vi "test Encode Parameters into Words for Labels in a Channel.vi"(8 "error in":errorcluster, 11 "TestCase in":refnum<class "Engine.lvclass">) -> (0 "error out":errorcluster, 3 "TestCase out":refnum<class "Engine.lvclass">)   [LabVIEW 2020, in "Engine.lvclass"]
uses:
  Engine.lvclass
  Shared/RT Label Settings.ctl
  Shared/Label.ctl
  Shared/RT Parameters.ctl
  Shared/Parameter Definition.ctl
  <vilib>/NI/NI VeriStand Encoding and Decoding/Encoding.ctl
  <vilib>/NI VeriStand/Custom Device API/Custom Device Item Ref.ctl
  Shared/Transfer Type.ctl
  <vilib>/NI VeriStand/Custom Device API/Data Reference.ctl
  <vilib>/addons/_JKI Toolkits/VI Tester/TestCase.llb/TestCase.lvclass
  <vilib>/NI VeriStand/Custom Device API/Custom Device API.lvlib
  <vilib>/NI/NI VeriStand Encoding and Decoding/Encoding and Decoding.lvlib
  Engine/Implementation/Tx Scheduled Labels Execution Unit/Tx Scheduled Labels Execution Unit.lvclass
  C:/Program Files (x86)/National Instruments/LabVIEW 2020/vi.lib/addons/_JKI Toolkits/VI Tester/TestCase.llb/TestCase.lvclass
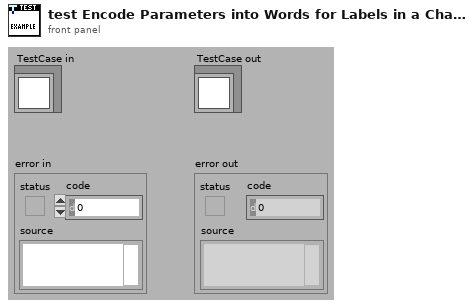
[diagram p1: front panel]
types:
  T1 = typedef "RT Label Settings.ctl" = cluster{"Name":string, "xmlName":string, "label":T2, "transfer period":u32, "SDI_Enabled":bool, "SDI":u8, "parameter driver data":T3, "transfer type":T7, "has timestamp?":bool, "Label Disable/Trigger Channel Reference":T6, "Message Handle":u64, "Initialized?":bool, "Word Initial Raw Value":u32, "Label Timestamp Channel Data Reference":T8, "disabled":bool}
  T2 = typedef "Label.ctl" = u8
  T3 = typedef "RT Parameters.ctl" = cluster{"parameter definitions":T4[], "Tx parameter refs":T6[]}
  T4 = typedef "Parameter Definition.ctl" = cluster{"start index":i32, "size":i32, "encoding":T5, "signed":bool, "scale multiplier":dbl, "scale offset":dbl, "default value":dbl}
  T5 = typedef "Encoding and Decoding.lvlib/Encoding.ctl" = enum16{"BNR", "BCD", "Discrete"}
  T6 = typedef "Custom Device API.lvlib/Custom Device Item Ref.ctl" = u64
  T7 = typedef "Transfer Type.ctl" = enum16{"Scheduled", "Acyclic", "Block", "Strobe"}
  T8 = typedef "Custom Device API.lvlib/Data Reference.ctl" = i32
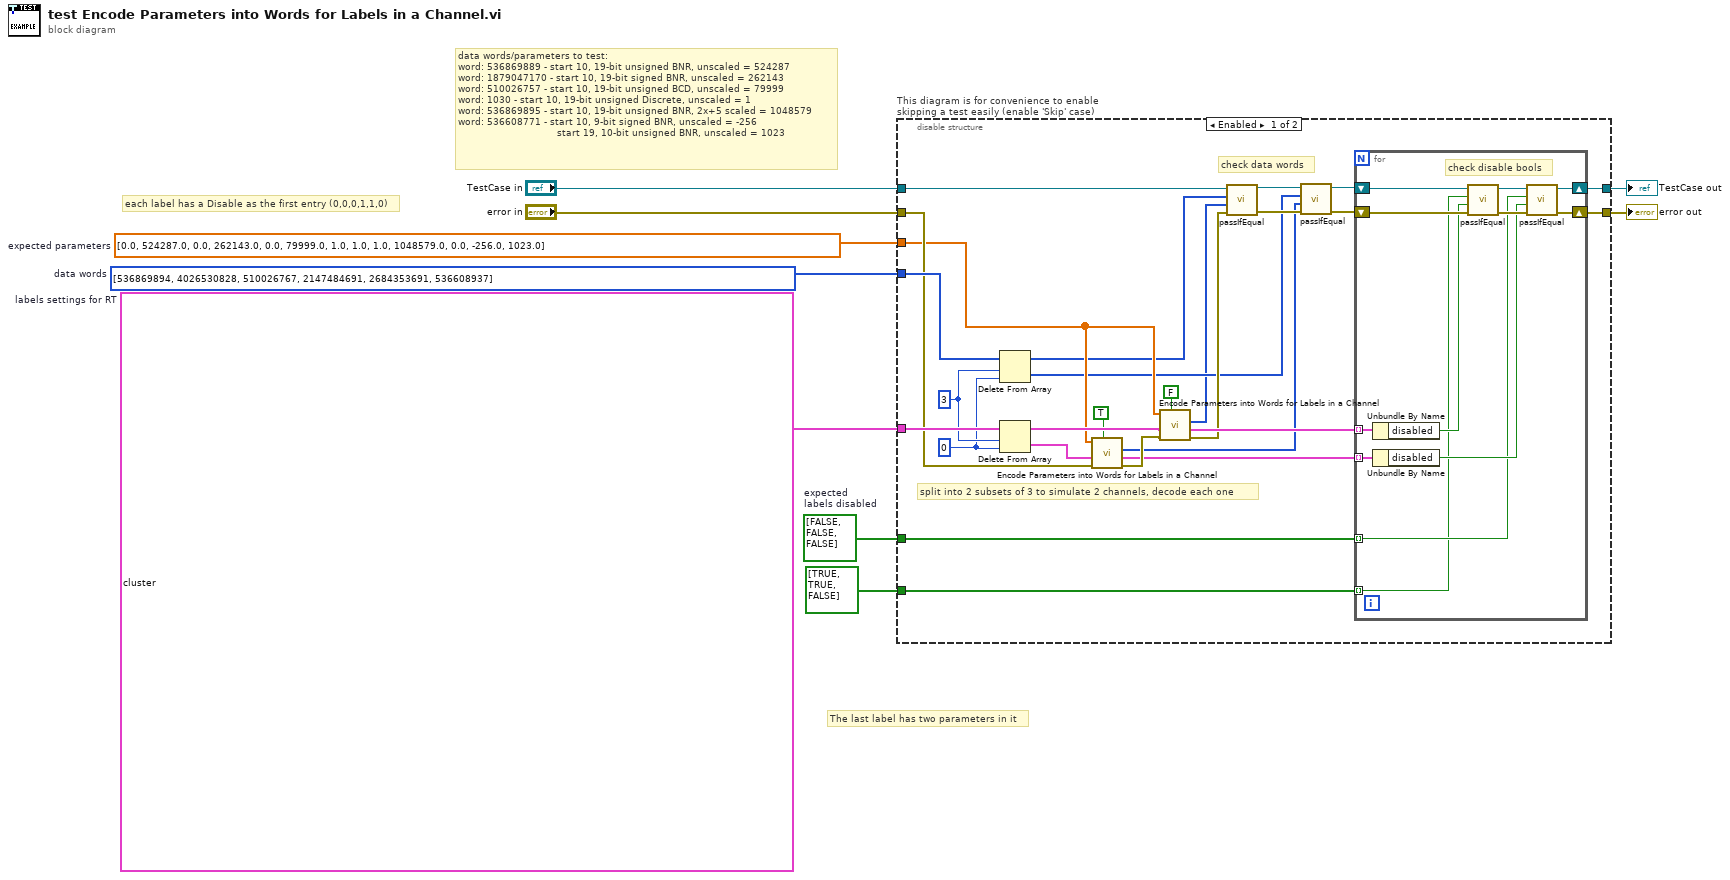
[diagram p0: block diagram]
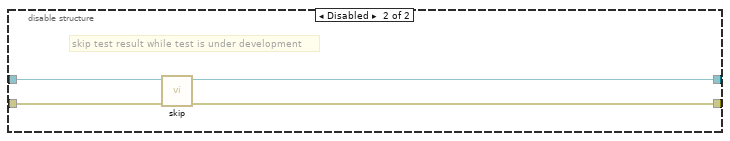
[diagram p2: hidden frame]
diagram:
  w2 = bool[] [FALSE, FALSE, FALSE]  # expected labels disabled
  w4 = dbl[] [0.0, 524287.0, 0.0, 262143.0, 0.0, 79999.0, 1.0, 1.0, 1.0, 1048579.0, 0.0, -256.0, 1023.0]  # expected parameters
  w5 = T1[] [{"Name"="", "xmlName"="", "label"=6, "transfer period"=10, "SDI_Enabled"=FALSE, "SDI"=0, "parameter driver data"={"parameter definitions"=[{"start index"=10, "size"=19, "encoding"=enum."BNR", "signed"=FALSE, "scale multiplier"=1.0, "scale offset"=0.0, "default value"=0.0}], "Tx parameter refs"=[]}, "transfer type"=enum."Scheduled", "has timestamp?"=FALSE, "Label Disable/Trigger Channel Reference"=0, "Message Handle"=0, "Initialized?"=FALSE, "Word Initial Raw Value"=0, "Label Timestamp Channel Data Reference"=0, "disabled"=FALSE}, {"Name"="", "xmlName"="", "label"=12, "transfer period"=10, "SDI_Enabled"=FALSE, "SDI"=0, "parameter driver data"={"parameter definitions"=[{"start index"=10, "size"=19, "encoding"=enum."BNR", "signed"=TRUE, "scale multiplier"=1.0, "scale offset"=0.0, "default value"=0.0}], "Tx parameter refs"=[]}, "transfer type"=enum."Scheduled", "has timestamp?"=FALSE, "Label Disable/Trigger Channel Reference"=0, "Message Handle"=0, "Initialized?"=FALSE, "Word Initial Raw Value"=0, "Label Timestamp Channel Data Reference"=0, "disabled"=FALSE}, {"Name"="", "xmlName"="", "label"=15, "transfer period"=10, "SDI_Enabled"=FALSE, "SDI"=0, "parameter driver data"={"parameter definitions"=[{"start index"=10, "size"=19, "encoding"=enum."BCD", "signed"=FALSE, "scale multiplier"=1.0, "scale offset"=0.0, "default value"=0.0}], "Tx parameter refs"=[]}, "transfer type"=enum."Scheduled", "has timestamp?"=FALSE, "Label Disable/Trigger Channel Reference"=0, "Message Handle"=0, "Initialized?"=FALSE, "Word Initial Raw Value"=0, "Label Timestamp Channel Data Reference"=0, "disabled"=FALSE}, {"Name"="", "xmlName"="", "label"=19, "transfer period"=10, "SDI_Enabled"=FALSE, "SDI"=0, "parameter driver data"={"parameter definitions"=[{"start index"=10, "size"=19, "encoding"=enum."Discrete", "signed"=FALSE, "scale multiplier"=1.0, "scale offset"=0.0, "default value"=0.0}], "Tx parameter refs"=[]}, "transfer type"=enum."Scheduled", "has timestamp?"=FALSE, "Label Disable/Trigger Channel Reference"=0, "Message Handle"=0, "Initialized?"=FALSE, "Word Initial Raw Value"=0, "Label Timestamp Channel Data Reference"=0, "disabled"=FALSE}, {"Name"="", "xmlName"="", "label"=155, "transfer period"=10, "SDI_Enabled"=FALSE, "SDI"=0, "parameter driver data"={"parameter definitions"=[{"start index"=10, "size"=19, "encoding"=enum."BNR", "signed"=FALSE, "scale multiplier"=2.0, "scale offset"=5.0, "default value"=0.0}], "Tx parameter refs"=[]}, "transfer type"=enum."Scheduled", "has timestamp?"=FALSE, "Label Disable/Trigger Channel Reference"=0, "Message Handle"=0, "Initialized?"=FALSE, "Word Initial Raw Value"=0, "Label Timestamp Channel Data Reference"=0, "disabled"=FALSE}, {"Name"="", "xmlName"="", "label"=169, "transfer period"=10, "SDI_Enabled"=FALSE, "SDI"=0, "parameter driver data"={"parameter definitions"=[{"start index"=10, "size"=9, "encoding"=enum."BNR", "signed"=TRUE, "scale multiplier"=1.0, "scale offset"=0.0, "default value"=0.0}, {"start index"=19, "size"=10, "encoding"=enum."BNR", "signed"=FALSE, "scale multiplier"=1.0, "scale offset"=0.0, "default value"=0.0}], "Tx parameter refs"=[]}, "transfer type"=enum."Scheduled", "has timestamp?"=FALSE, "Label Disable/Trigger Channel Reference"=0, "Message Handle"=0, "Initialized?"=FALSE, "Word Initial Raw Value"=0, "Label Timestamp Channel Data Reference"=0, "disabled"=FALSE}]  # labels settings for RT
  w6 = u32[] [536869894, 4026530828, 510026767, 2147484691, 2684353691, 536608937]  # data words
  # "each label has a Disable as the first entry (0,0,0,1,1,0)"
  # "The last label has two parameters in it"
  # "for visibility, irrelevant label settings are minimized in this constant"
  # "data words/parameters to test:\nword: 536869889 - start 10, 19-bit unsigned BNR, unscaled = 524287\nword: 1879047170 - start 10, 19-bit signed BNR, unscaled = 262143\nword: 510026757 - start 10, 19-bit unsigned BCD, unscaled = 79999\nword: 1030 - start 10, 19-bit unsigned Discrete, unscaled = 1\nword: 536869895 - start 10, 19-bit unsigned BNR, 2x+5 scaled = 1048579 \nword: 536608771 - start 10, 9-bit signed BNR, unscaled = -256\n                                 start 19, 10-bit unsigned BNR, unscaled = 1023"
  n1 = disable-structure "This diagram is for convenience to enable skipping a test easily (enable 'Skip' case)" shown="Enabled" {
    disable-tunnel: "TestCase in" -> [w34 w52]
    disable-tunnel: [w25 w50] -> w3
    disable-tunnel: [w24 w51] -> w8
    disable-tunnel: "error in" -> [w30 w49]
    disable-tunnel: w6 -> [w35 _]
    disable-tunnel: w5 -> [w36 _]
    disable-tunnel: w4 -> [w26 _]
    disable-tunnel: w2 -> [w21 _]
    disable-tunnel: bool[] [TRUE, TRUE, FALSE] -> [w20 _]
    frame Enabled {
      w32 = 0 ("index")
      w33 = 3 ("length")
      # "check data words"
      # "split into 2 subsets of 3 to simulate 2 channels, decode each one"
      n2 = Delete From Array(array=w35, length=w33, index=w32) -> (deleted portion=w13:u32[], array with subset deleted=w12:u32[])
      n3 = Delete From Array(array=w36, length=w33, index=w32) -> (deleted portion=w31:T1[], array with subset deleted=w28:T1[])
      n4 = call "Encode Parameters into Words for Labels in a Channel.vi"("reset index"=TRUE, "error in (no error)"=w30, "labels settings for RT in"=w31, "Parameter Values in"=w26) -> ("error out"=w27:errorcluster, "labels settings for RT out"=w23:T1[], "data words out"=w14:u32[])  [unwired: 5 in]
      n5 = call "Encode Parameters into Words for Labels in a Channel.vi"("reset index"=FALSE, "error in (no error)"=w27, "labels settings for RT in"=w28, "Parameter Values in"=w26) -> ("error out"=w19:errorcluster, "labels settings for RT out"=w22:T1[], "data words out"=w11:u32[])  [unwired: 5 in]
      n6 = call-dynamic "passIfEqual.vi"("error in (no error)"=w19, "y"=w11, "x"=w12, "TestCase in"=w34) -> ("error out"=w15:errorcluster, "TestCase out"=w16:refnum<class "Engine.lvclass">)  [unwired: 6 in]
      n7 = call-dynamic "passIfEqual.vi"("error in (no error)"=w15, "y"=w14, "x"=w13, "TestCase in"=w16) -> ("error out"=w18:errorcluster, "TestCase out"=w17:refnum<class "Engine.lvclass">)  [unwired: 6 in]
      n8 = for {
        shift-right: [w41] -> w25
        shift-left: w17 -> [w48]
        shift-right: [w40] -> w24
        shift-left: w18 -> [w47]
        tunnel: w23 -> [w45] mode=indexing
        tunnel: w22 -> [w46] mode=indexing
        tunnel: w21 -> [w38] mode=indexing
        tunnel: w20 -> [w37] mode=indexing
        # "check disable bools"
        n9 = Unbundle By Name(w46) -> ("disabled"=w44:bool)
        n10 = Unbundle By Name(w45) -> ("disabled"=w39:bool)
        n11 = call-dynamic "passIfEqual.vi"("error in (no error)"=w47, "y"=w44, "x"=w37, "TestCase in"=w48) -> ("error out"=w42:errorcluster, "TestCase out"=w43:refnum<class "Engine.lvclass">)  [unwired: 6 in]
        n12 = call-dynamic "passIfEqual.vi"("error in (no error)"=w42, "y"=w39, "x"=w38, "TestCase in"=w43) -> ("error out"=w40:errorcluster, "TestCase out"=w41:refnum<class "Engine.lvclass">)  [unwired: 6 in]
      }
    }
    frame Disabled {
      # "skip test result while test is under development"
      n13 = call <vilib>:"skip.vi"("error in (no error)"=w49, "TestCase in"=w52) -> ("error out"=w51:errorcluster, "TestCase out"=w50:refnum<class "Engine.lvclass">)  [unwired: 8 in]
    }
  }
  "error out" <- w8
  "TestCase out" <- w3
